vi "Configure Current.vi"(0 "VISA resource name":refnum<visa-resource-name>, 5 "Current Level (0 A)":dbl, 7 "Enable Current Protection (Enabled)":bool=TRUE, 9 "Current Protection Delay (0.1 Sec)":dbl=0.1, 11 "error in (no error)":errorcluster) -> (4 "VISA resource name out":refnum<visa-resource-name>, 15 "error out":errorcluster)   [LabVIEW 2013, in "Cal Inst.lvlib" / "California Instruments iX Series.lvlib"]
doc: "Configures the output current of the AC source and also the current protection."
uses:
  California Instruments iX Series.lvlib
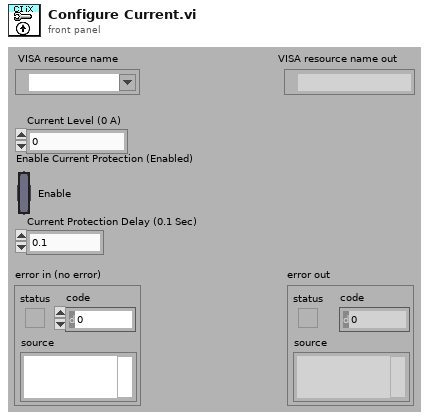
[diagram p1: front panel]
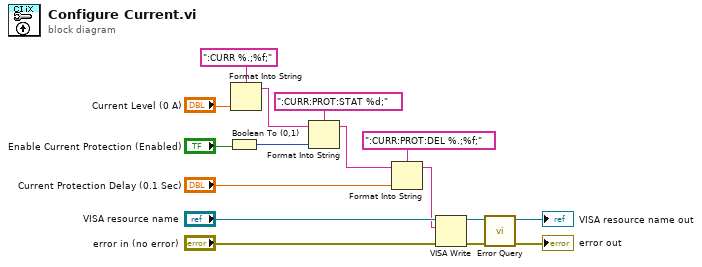
[diagram p0: block diagram]
diagram:
  n1 = Boolean To (0,1)(Boolean="Enable Current Protection (Enabled)") -> (0, 1=w6:i16)
  n2 = Format Into String(format string=":CURR %.;%f;", "Current Level (0 A)") -> (resulting string=w8:string)  [unwired: 2 in, 1 out]
  n3 = Format Into String(format string=":CURR:PROT:STAT %d;", initial string=w8, w6) -> (resulting string=w4:string)  [unwired: 1 in, 1 out]
  n4 = Format Into String(format string=":CURR:PROT:DEL %.;%f;", initial string=w4, "Current Protection Delay (0.1 Sec)") -> (resulting string=w1:string)  [unwired: 1 in, 1 out]
  n5 = VISA Write(VISA resource name="VISA resource name", write buffer=w1, error in (no error)="error in (no error)") -> (VISA resource name out=w14:refnum<visa-resource-name>, error out=w13:errorcluster)  [unwired: 1 out]
  n6 = call "Error Query.vi"("error in (no error)"=w13, "VISA resource name"=w14) -> ("error out"=→"error out":errorcluster, "VISA resource name out"=→"VISA resource name out":refnum<visa-resource-name>)  [unwired: 6 in, 2 out]
